vi "unused_test_stackInGrid.vi"(11 "Test Case In":refnum<class "StackTests.lvclass">) -> (0 "error out":errorcluster, 3 "Test Case Out":refnum<class "StackTests.lvclass">)   [LabVIEW 2023]
uses:
  StackTests.lvclass/StackTests.ctl
  <vilib>/Astemes/LUnit/Test Case.lvclass
  source/direction.ctl
  source/TLC_Geometry.lvlib
  source/alignment.ctl
  StackTests.lvclass
  C:/Program Files (x86)/National Instruments/LabVIEW 2023/vi.lib/Astemes/LUnit/Test Case.lvclass
  C:/Program Files (x86)/National Instruments/LabVIEW 2023/vi.lib/Astemes/LUnit/LUnit Runnable.lvclass
  C:/projects/TLC_Geometry/tests/StackTests/StackTests.lvclass
panel:
  in  "Numeric 2":dbl
  in  "btn 2":bool
  in  "firstItem 2":string
  in  "String 2":string
  in  "Numeric":dbl
  in  "btn":bool
  in  "firstItem":string
  in  "String":string
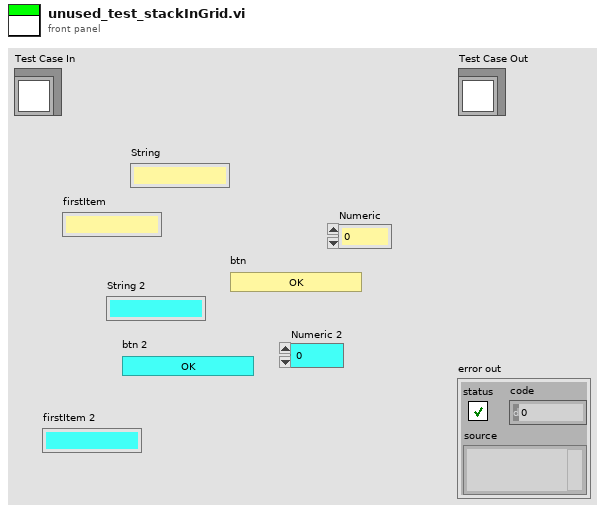
[diagram p1: front panel]
types:
  T1 = typedef "TLC_Geometry.lvlib/alignment.ctl" = enum16{"None", "AlignTop", "AlignBottom", "AlignHorizontalCenters", "AlignLeft", "AlignRight", "AlignVerticalCenters"}
  T2 = typedef "TLC_Geometry.lvlib/direction.ctl" = enum16{"Horizontally", "Vertically"}
  T3 = typedef "LVPositionTypeDef.ctl" = cluster{"Left":i32, "Top":i32}
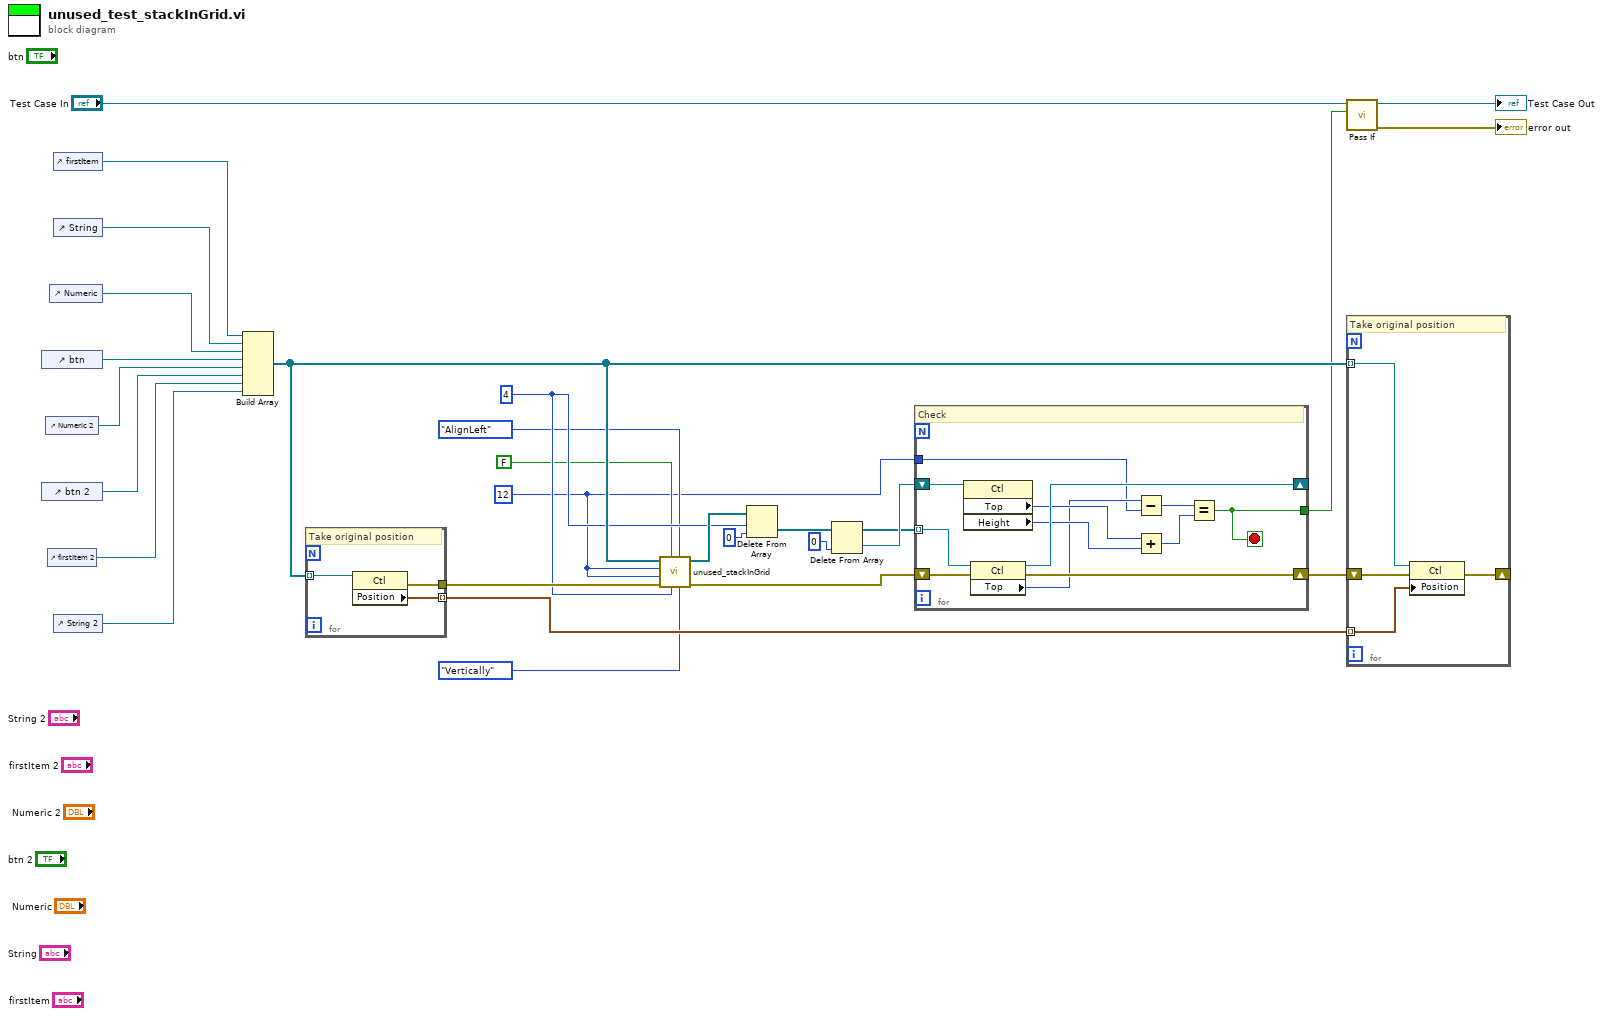
[diagram p0: block diagram]
diagram:
  w6 = 4 ("elementsInPreferredDirection")
  w1 = u16 12 ("spacing")
  n1 = control-ref of="btn"() -> (w13:refnum<vi>)
  n2 = control-ref of="btn 2"() -> (w11:refnum<vi>)
  n3 = control-ref of="Numeric 2"() -> (w12:refnum<vi>)
  n4 = control-ref of="firstItem 2"() -> (w10:refnum<vi>)
  n5 = control-ref of="Numeric"() -> (w14:refnum<vi>)
  n6 = control-ref of="firstItem"() -> (w25:refnum<vi>)
  n7 = control-ref of="String"() -> (w24:refnum<vi>)
  n8 = control-ref of="String 2"() -> (w9:refnum<vi>)
  n9 = Build Array(w25, w24, w14, w13, w12, w11, w10, w9) -> (w17:refnum<vi>[])
  n10 = for {
    tunnel: w17 -> [w31] mode=indexing
    tunnel: [w30] -> w15 mode=indexing
    tunnel: [w29] -> w23
    # "Take original position"
    n11 = property class="Ctl"(reference=w31) -> (error out=w29:errorcluster, "Position"=w30:T3)  [unwired: 1 in, 1 out]
  }
  n12 = call "unused_stackInGrid.vi"("preferredDirection"=direction."Vertically", "alignmentInTheSecondaryDirection"=alignment."AlignLeft", "elementsInPreferredDirection"=w6, "useControlBodyOnly"=FALSE, "error in (no error)"=w23, "horizontalSpacing"=w1, "verticalSpacing"=w1, "refs"=w17) -> ("error out"=w22:errorcluster, "refs(dup)"=w7:refnum<vi>[])  [unwired: 2 in]
  n13 = Delete From Array(array=w7, length=w6, index=0) -> (deleted portion=w4:refnum<vi>[])  [unwired: 1 out]
  n14 = Delete From Array(array=w4, index=0) -> (deleted portion=w20:refnum<vi>, array with subset deleted=w19:refnum<vi>[])  [unwired: 1 in]
  n15 = for {
    tunnel: w19 -> [w43] mode=indexing
    shift-right: [w41] -> w18
    shift-left: w22 -> [w42]
    shift-right: [w39] -> _
    shift-left: w20 -> [w40]
    tunnel: [w35] -> w16
    tunnel: w1 -> [w32]
    stop <- w35 stop-if-true
    # "Check"
    n16 = property class="Ctl"(reference=w40) -> ("Top"=w38:i32, "Height"=w37:u32)  [unwired: 1 in, 2 out]
    n17 = property class="Ctl"(reference=w43, error in=w42) -> (reference out=w39:refnum<vi>, error out=w41:errorcluster, "Top"=w34:i32)
    n18 = Subtract(x=w34, y=w32) -> (x-y=w33:i32)
    n19 = Add(x=w38, y=w37) -> (x+y=w36:u32)
    n20 = Equal?(x=w33, y=w36) -> (x = y?=w35:bool)
  }
  n21 = call <vilib>:"Pass If.vi"("Pass?"=w16, "LUnit Test Case In"="Test Case In") -> ("error out"=→"error out":errorcluster, "LUnit Test Case Out"=→"Test Case Out":refnum<class "StackTests.lvclass">)  [unwired: 8 in]
  n22 = for {
    tunnel: w17 -> [w47] mode=indexing
    tunnel: w15 -> [w46] mode=indexing
    shift-right: [w45] -> _
    shift-left: w18 -> [w44]
    # "Take original position"
    n23 = property class="Ctl"(reference=w47, error in=w44, "Position"=w46) -> (error out=w45:errorcluster)  [unwired: 1 out]
  }
